vi "Image_Display_RAW12_U16.vi"(6 "Scale by Power of 2":i16=4, 7 "Bayer Pattern":T2, 8 "error in (no error)":errorcluster, 9 "Image Name":string="RAW12_U16", 10 "Image Configuration":T1={"Width"=1920, "Height"=1080}, 11 "RAW12_U16":u16[](array[numeric])) -> (0 "error out":errorcluster, 1 "Image":T3(plugin-control), 2 "Image Configuration Out":T1, 3 "RGB Frame Out":u8[](array[numeric]))   [LabVIEW 2020]
uses:
  ctl/Image_Configuration.ctl
  ctl/Image_RAW_Bayer_Pattern.ctl
  <vilib>/vision/Image Controls.llb/IMAQ Image.ctl
  <vilib>/vision/EDVR.llb/IMAQ ImageToEDVR 2D U16.vi
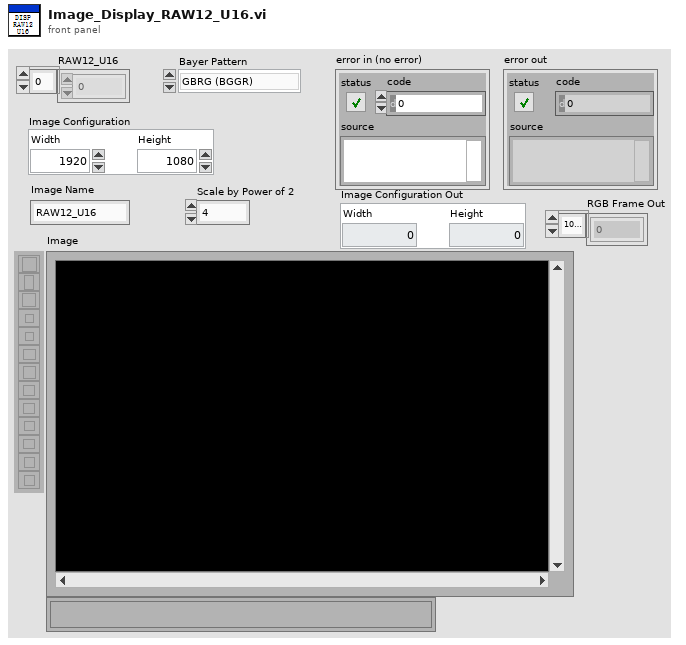
[diagram p1: front panel]
types:
  T1 = typedef "Image_Configuration.ctl" = cluster{"Width":i32, "Height":i32}
  T2 = typedef "Image_RAW_Bayer_Pattern.ctl" = enum16{"GBRG (BGGR)", "GRBG (RGGB)", "BGGR (GBRG)", "RGGB (GRBG)", "CRBC (RCCB)"}
  T3 = typedef "IMAQ Image.ctl" = refnum<image>
  T4 = cluster{"Pattern":i32, "Algorithm":i32, "Red Gain":dbl, "Green Gain":dbl, "Blue Gain":dbl}
  T5 = typedef "Image Type" = u32
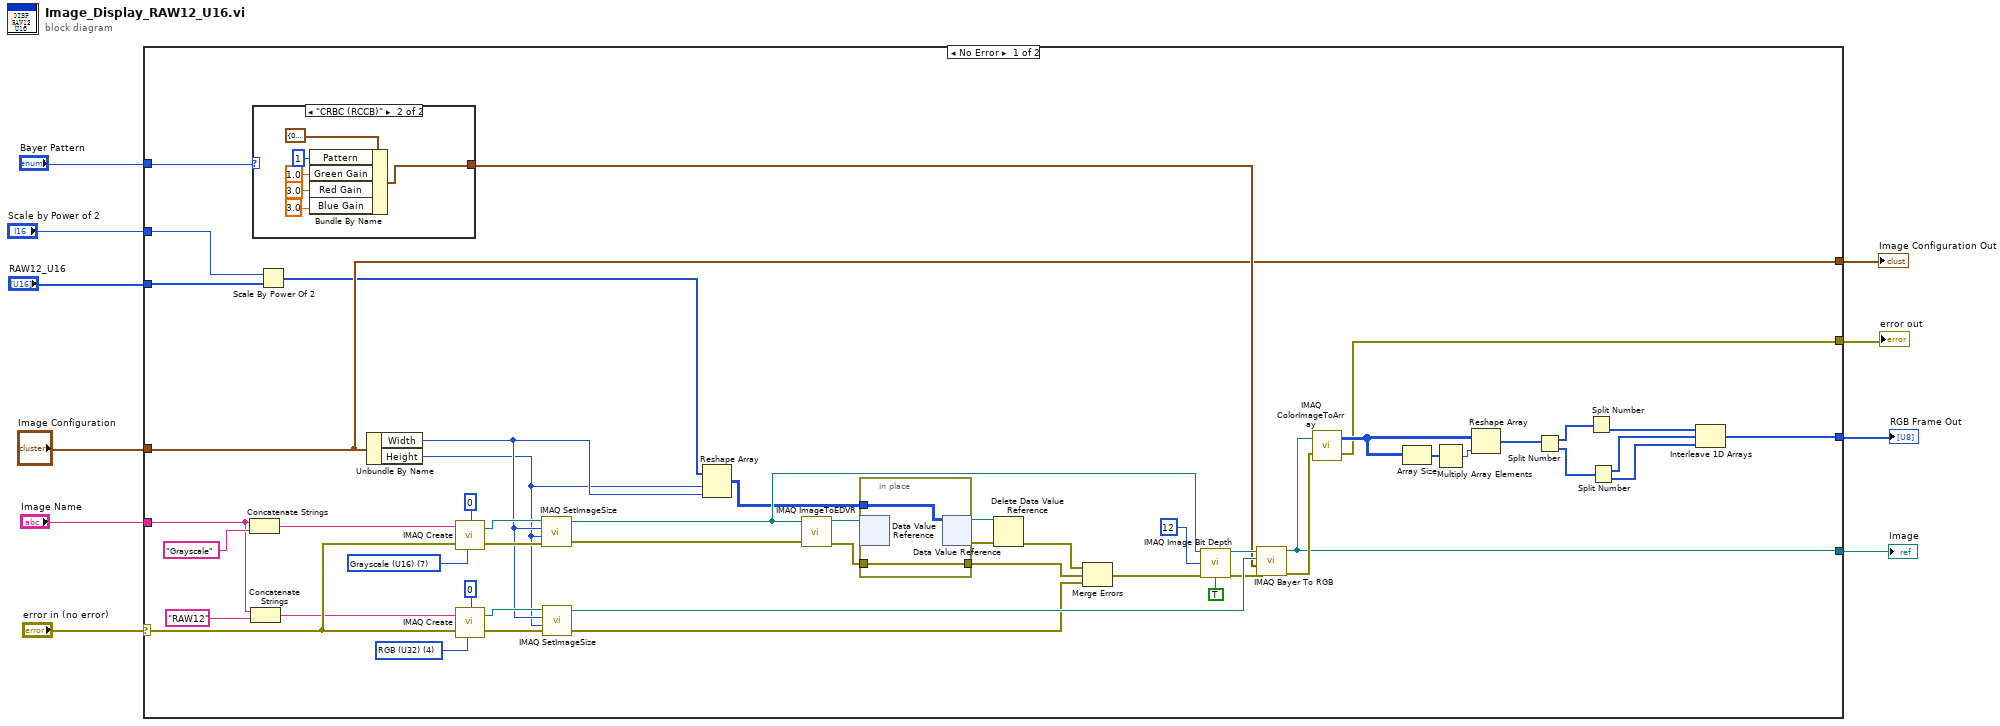
[diagram p0: block diagram]
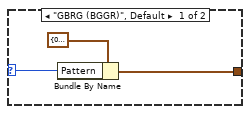
[diagram p2: hidden frame]
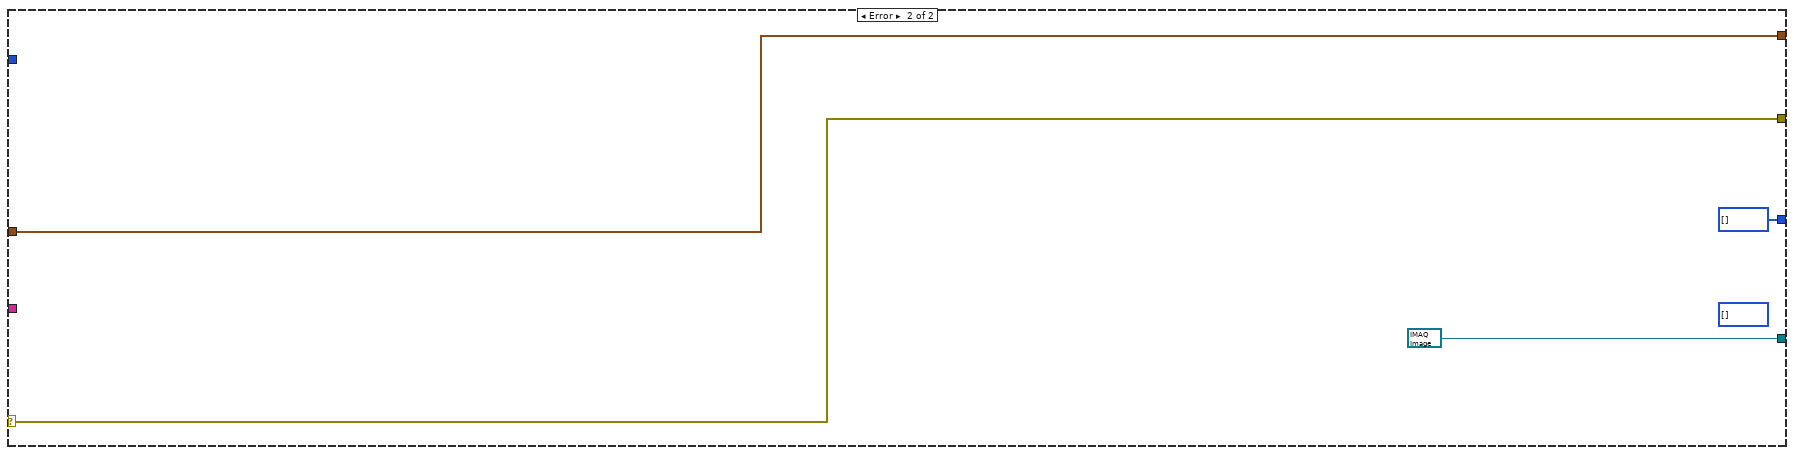
[diagram p3: hidden frame]
diagram:
  n1 = case shown="No Error" "error in (no error)" {
    selector: "error in (no error)" -> [w46 w76]
    tunnel: [w11 w76] -> w9
    tunnel: [w22 T3 refnum ("Image")] -> w8
    tunnel: "Image Configuration" -> [w26 w74]
    tunnel: "RAW12_U16" -> [w25 _]
    tunnel: "Image Name" -> [w34 _]
    tunnel: "Bayer Pattern" -> [w32 _]
    tunnel: [w12 u8[] []] -> w3
    tunnel: [w26 w74] -> w2
    tunnel: "Scale by Power of 2" -> [w23 _]
    frame No Error {
      w58 = T5 4 items=["Grayscale (U8)", "Grayscale (I16)", "Grayscale (SGL)", "Complex (CSG)", "RGB (U32)", "HSL (U32)", "RGB (U64)", "Grayscale (U16)"] ("Image Type")
      w60 = T5 7 items=["Grayscale (U8)", "Grayscale (I16)", "Grayscale (SGL)", "Complex (CSG)", "RGB (U32)", "HSL (U32)", "RGB (U64)", "Grayscale (U16)"] ("Image Type")
      n2 = Concatenate Strings(w34, "Grayscale" ("Image Name")) -> (w36:string)
      n3 = Concatenate Strings(w34, "RAW12" ("Image Name")) -> (w33:string)
      n4 = case shown="\"CRBC (RCCB)\"" w32 {
        selector: w32 -> [w63 _]
        tunnel: [w62 w65] -> w31
        frame "GBRG (BGGR)", Default {
          n5 = Bundle By Name(cluster=T4 {"Pattern"=0, "Algorithm"=0, "Red Gain"=1.0, "Green Gain"=1.0, "Blue Gain"=1.0} ("Bayer Parameters"), "Pattern"=w63) -> (w62:T4)
        }
        frame "CRBC (RCCB)" {
          n6 = Bundle By Name(cluster=T4 {"Pattern"=0, "Algorithm"=0, "Red Gain"=1.0, "Green Gain"=1.0, "Blue Gain"=1.0} ("Bayer Parameters"), "Pattern"=1, "Green Gain"=1.0, "Red Gain"=3.0, "Blue Gain"=3.0) -> (w65:T4)
        }
      }
      n7 = Scale By Power Of 2(n=w23, x=w25) -> (x*2^n=w24:u16[])
      n8 = Unbundle By Name(w26) -> ("Width"=w30:i32, "Height"=w29:i32)
      n9 = call "IMAQ Create"("Border Size"=0, "Image Name"=w36, "Image Type"=w60, "error in (no error)"=w46) -> ("New Image"=w56:T3, "error out"=w57:errorcluster)  [unwired: 1 in]
      n10 = call "IMAQ Create"("Border Size"=0, "Image Name"=w33, "Image Type"=w58, "error in (no error)"=w46) -> ("New Image"=w54:T3, "error out"=w55:errorcluster)  [unwired: 1 in]
      n11 = call "IMAQ SetImageSize"("error in (no error)"=w57, "Y Resolution"=w29, "X Resolution"=w30, "Image"=w56) -> ("error out"=w45:errorcluster, "Image Out"=w38:T3)  [unwired: 1 in]
      n12 = call "IMAQ SetImageSize"("error in (no error)"=w55, "Y Resolution"=w29, "X Resolution"=w30, "Image"=w54) -> ("error out"=w48:errorcluster, "Image Out"=w50:T3)  [unwired: 1 in]
      n13 = Reshape Array(w24, w29, w30) -> (w28:u16[][])
      n14 = call-poly <vilib>:"IMAQ ImageToEDVR.vi"("error out"=w45, "Image"=w38) -> ("error out"=w43:errorcluster, "EDVR 2D U16"=w44:refnum<data-value>)  [unwired: 7 in, 1 out]
      n15 = in-place {
        in-place-border: w43 -> [w72]
        in-place-border: [w72] -> w42
        in-place-border: w28 -> [w71]
        n16 = in-place-dvr #1(w44) -> ()  [unwired: 2 out]
        n17 = in-place-dvr #1(w71) -> (w41:refnum<data-value>, w40:errorcluster)
      }
      n18 = Delete Data Value Reference(data value reference=w41, error in=w40) -> (error out=w39:errorcluster)  [unwired: 1 out]
      n19 = Merge Errors(w39, w42, w48) -> (w47:errorcluster)
      n20 = call "IMAQ Image Bit Depth"("Image"=w38, "Bit Depth (0)"=u32 12, "error in (no error)"=w47, "Get/Set Bit Depth? (Set)"=TRUE) -> ("Image Out"=w51:T3, "error out"=w49:errorcluster)  [unwired: 9 in, 1 out]
      n21 = call "IMAQ Bayer To RGB"("error in (no error)"=w49, "Bayer Parameters"=w31, "Image Dst"=w50, "Image Src"=w51) -> ("error out"=w27:errorcluster, "Image Dst Out"=w22:T3)  [unwired: 6 in]
      n22 = call "IMAQ ColorImageToArray"("Image"=w22, "error in (no error)"=w27) -> ("Image Pixels (U32)"=w13:u32[][], "error out"=w11:errorcluster)  [unwired: 2 in, 1 out]
      n23 = Array Size(array=w13) -> (size(s)=w21:i32[])
      n24 = Multiply Array Elements(1:w21) -> (0:w20:i32)
      n25 = Reshape Array(w13, w20) -> (w19:u32[])
      n26 = Split Number(x=w19) -> (hi(x)=w18:u16[], lo(x)=w17:u16[])
      n27 = Split Number(x=w18) -> (lo(x)=w14:u8[])  [unwired: 1 out]
      n28 = Split Number(x=w17) -> (hi(x)=w16:u8[], lo(x)=w15:u8[])
      n29 = Interleave 1D Arrays(w14, w16, w15) -> (w12:u8[])
    }
    frame Error {
      (unwired) u8[] []
    }
  }
  "error out" <- w9
  "Image" <- w8
  "RGB Frame Out" <- w3
  "Image Configuration Out" <- w2
